vi "Cache.Result.ComponentGet.vi"(7 "Idx":i32, 8 "error in (no error)":errorcluster, 10 "ProdComp in":T1) -> (0 "error out":errorcluster, 1 "Found":bool, 2 "ProdComp out":T1)   [LabVIEW 2016]
uses:
  Cache.ProductComponent.Data.ctl
  Tools/EventLog/EventLog.EventSource.ctl
  Tools/Translator/Translator.Message.ctl
  Tools/EventLog/EventLog.EventLevel.ctl
  Tools/EventLog/EventLog.New(array).vi
  Global/ApplicationGlobal.vi
  Tools/EventLog/EventLog.Buffer.vi
  Tools/EventLog/EventLog.File.ReadWrite.vi
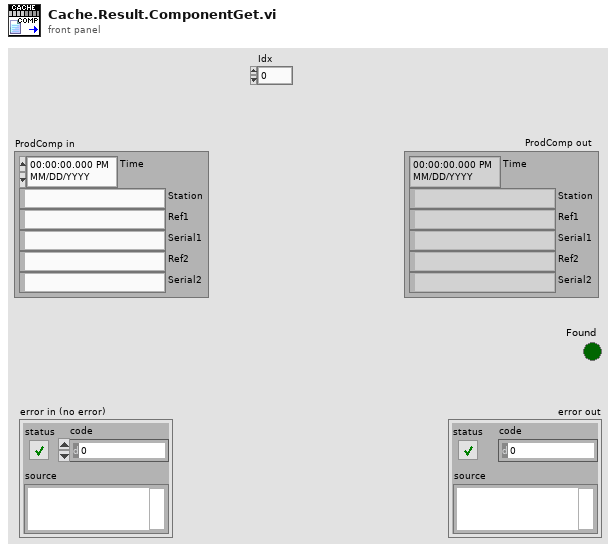
[diagram p1: front panel]
types:
  T1 = typedef "Cache.ProductComponent.Data.ctl" = cluster{"Time":timestamp, "Station":string, "Ref1":string, "Serial1":string, "Ref2":string, "Serial2":string}
  T2 = typedef "EventLog.EventLevel.ctl" = enum8{"Debug", "Info", "Warning", "Error"}
  T3 = typedef "Translator.Message.ctl" = enum16{"-", "Event confirmed", "Log out", "Log in", "Shutdown", "Cancel", "Start", "Continue", "Stop", "On", "Off", "OK", "NOK", "NOK %s", "This", "Prev", "Home", "Work", "In progress...", "Missing", "Empty", "Hardware failure", "Initial", "Error %d >> %s", "Error %d >> %s >> %s", "Starting %s", "Quitting %s", "Configured", "Initializing", "Quitting", "Loading", "Running %s", "Stopped", "Summary", "Do you want to continue?", "Do you want to exit?", "Log out?", "System", "All", "IDLE", "Translating...%s", "Not found", "Alarm %s", "Run", "Skip", "Abort", "Repeat", "Please wait...", "Database disconnected", "Login to database successful", "Login to database failed: %d; %s", "Get process step data for %s", "Changeover off", "Changeover into %s", "Product %s | %s found in cache with status %d at previous station", "Product %s | %s found in database with status %d at previous station", "Product %s | %s not found in cache at previous station", "Product %s | %s not found in database at previous station", "Product %s | %s found in cache with status %d at this station (%d repetion)", "Product %s | %s found in database with status %d at this station (%d repetition)", "Product %s | %s not found in cache at this station", "Product %s | %s not found in database at this station", "Product %s | %s found in cache for component %s | %s", "Product %s | %s found in database for component %s | %s", "Product not found in cache for component %s | %s", "Product not found in database for component %s | %s", "Product %s | %s connected with component %s | %s (cache)", "Product %s | %s connected with component %s | %s (database)", "New data for %s | %s (cache)", "New data for %s | %s (database)", "File %s moved (cache)", "File %s deleted (cache)", "Msg %d >> %s", "PLC LifeBit Failure", "Reconnecting DB", "Reconnecting PLC", "Free disk space is below 1GB - contact technician", "Unable to check product status", "Product %s SN %s checked in DB"}
  T4 = typedef "EventLog.EventSource.ctl" = enum16{"All", "Gui", "Cache", "PLC1", "PLC2", "PLC3", "DB", "DB01", "DB02", "DB03", "DB04", "DB05", "DB06", "DB07", "DB08", "DB09", "DB10", "DB11", "DB12", "DB13", "DB14", "DB15", "DB16"}
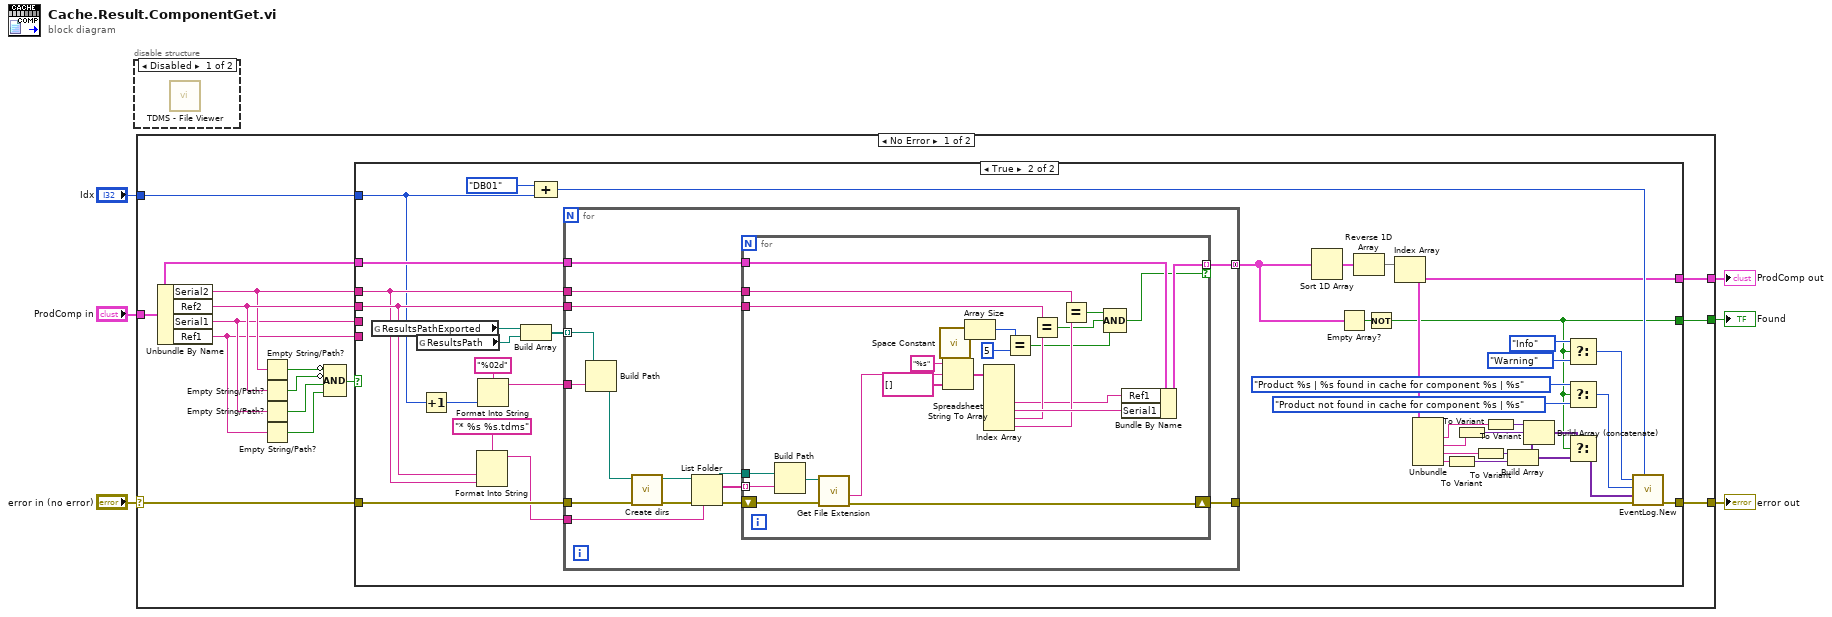
[diagram p0: block diagram]
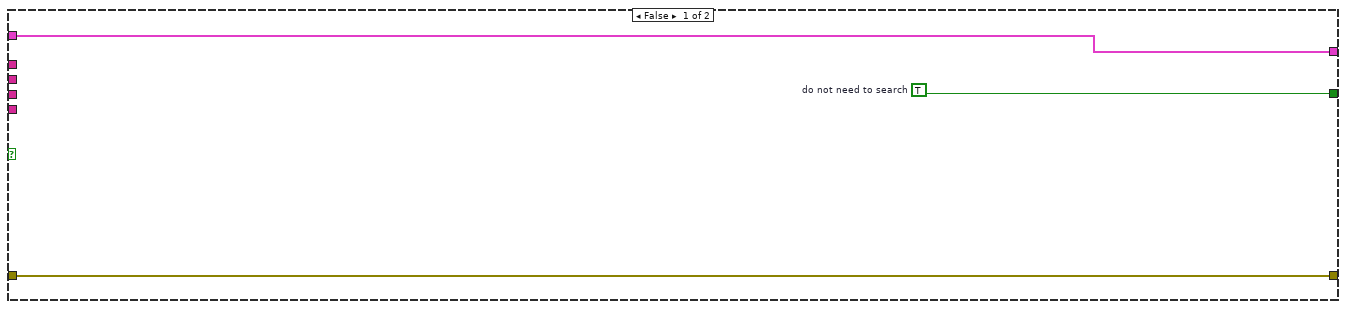
[diagram p2: hidden frame]
diagram:
  n1 = disable-structure shown="Disabled" {
    frame Disabled {
      n2 = call <vilib>:"TDMS - File Viewer.vi"() -> ()  [unwired: 6 in, 2 out]
    }
    frame Enabled {
    }
  }
  n3 = case shown="No Error" "error in (no error)" {
    selector: "error in (no error)" -> [w9 w104]
    tunnel: [w21 w104] -> w6
    tunnel: "ProdComp in" -> [w11 w103]
    tunnel: [w10 w103] -> w3
    tunnel: [w8 _] -> w2
    tunnel: "Idx" -> [w7 _]
    frame No Error {
      n4 = Unbundle By Name(w11) -> ("Serial2"=w19:string, "Ref2"=w20:string, "Serial1"=w18:string, "Ref1"=w17:string)
      n5 = Empty String/Path?(string/path=w19) -> (empty?=w16:bool)
      n6 = Empty String/Path?(string/path=w20) -> (empty?=w15:bool)
      n7 = Empty String/Path?(string/path=w18) -> (empty?=w14:bool)
      n8 = Empty String/Path?(string/path=w17) -> (empty?=w13:bool)
      n9 = Compound Arithmetic op=AND(invert w16, invert w15, w14, w13) -> (w12:bool)
      n10 = case shown="True" w12 {
        tunnel: [w24 w56] -> w21
        tunnel: w9 -> [w24 w63]
        tunnel: w20 -> [_ w34]
        tunnel: w19 -> [_ w33]
        tunnel: w18 -> [_ _]
        tunnel: w17 -> [_ _]
        tunnel: w11 -> [w23 w64]
        tunnel: [w23 w52] -> w10
        tunnel: [w22 w39] -> w8
        tunnel: w7 -> [_ w26]
        frame False {
          w22 = TRUE  # do not need to search
        }
        frame True {
          n11 = global read "ApplicationGlobal.vi" "ResultsPathExported"() -> (w32:path)
          n12 = global read "ApplicationGlobal.vi" "ResultsPath"() -> (w31:path)
          n13 = Increment(x=w26) -> (x+1=w25:i32)
          n14 = Format Into String(format string="* %s %s.tdms", w34, w33) -> (resulting string=w27:string)  [unwired: 2 in, 1 out]
          n15 = Format Into String(format string="%02d", w25) -> (resulting string=w28:string)  [unwired: 2 in, 1 out]
          n16 = Build Array(w32, w31) -> (w30:path[])
          n17 = Compound Arithmetic op=ADD(EventLog.EventSource."DB01" ("Source (All)"), w26) -> (w55:i32)
          n18 = for {
            tunnel: [w67] -> w57
            tunnel: w33 -> [w66]
            tunnel: w34 -> [w65]
            tunnel: w64 -> [w78]
            tunnel: w63 -> [w74]
            tunnel: w30 -> [w76] mode=indexing
            tunnel: [w77] -> w60 mode=concatenating
            tunnel: w28 -> [w75]
            tunnel: w27 -> [w72]
            n19 = Build Path(base path=w76, name or relative path=w75) -> (appended path=w69:path)
            n20 = call "Create dirs.vi"("error in (no error)"=w74, "deepest dir"=w69) -> ("error"=w73:errorcluster)  [unwired: 9 in]
            n21 = List Folder(path=w69, pattern=w72, error in=w73) -> (path out=w68:path, filenames=w70:string[], error out=w71:errorcluster)  [unwired: 1 in, 1 out]
            n22 = for {
              tunnel: w78 -> [w102]
              tunnel: [w101] -> w77 mode=indexing if=w81
              tunnel: w68 -> [w99]
              tunnel: w70 -> [w98] mode=indexing
              shift-right: [w96] -> w67
              shift-left: w71 -> [w100]
              tunnel: w66 -> [w79]
              tunnel: w65 -> [w80]
              n23 = Build Path(base path=w99, name or relative path=w98) -> (appended path=w97:path)
              n24 = call <vilib>:"Get File Extension.vi"("error in (no error)"=w100, "file"=w97) -> ("error out"=w96:errorcluster, "filename without extension"=w95:string)  [unwired: 5 in, 3 out]
              n25 = call <vilib>:"Space Constant.vi"() -> ("String"=w92:string)
              n26 = Spreadsheet String To Array(delimiter (Tab)=w92, format string="%s", spreadsheet string=w95, array type (2D Dbl)=string[] []) -> (array=w90:string[])
              n27 = Array Size(array=w90) -> (size(s)=w89:i32)
              n28 = Index Array(array=w90) -> (element #3=w85:string, element #4=w91:string, element #5=w87:string, element #6=w86:string)  [unwired: 6 in, 2 out]
              n29 = Equal?(x=w89, y=5) -> (x = y?=w82:bool)
              n30 = Equal?(x=w80, y=w87) -> (x = y?=w83:bool)
              n31 = Equal?(x=w79, y=w86) -> (x = y?=w84:bool)
              n32 = Compound Arithmetic op=AND(w84, w83, w82) -> (w81:bool)
              n33 = Bundle By Name(cluster=w102, "Ref1"=w85, "Serial1"=w91) -> (w101:T1)
            }
          }
          n34 = Sort 1D Array(array=w60) -> (sorted array=w62:T1[])
          n35 = Empty Array?(array=w60) -> (empty?=w59:bool)
          n36 = Reverse 1D Array(array=w62) -> (reversed array=w61:T1[])
          n37 = Not(x=w59) -> (.not. x?=w39:bool)
          n38 = Index Array(array=w61) -> (element=w52:T1)  [unwired: 1 in]
          n39 = Unbundle(w52) -> ("Ref1"=w37:string, "Serial1"=w38:string, "Ref2"=w50:string, "Serial2"=w51:string)  [unwired: 2 out]
          n40 = To Variant(anything=w51) -> (Variant=w47:variant)
          n41 = To Variant(anything=w38) -> (Variant=w54:variant)
          n42 = To Variant(anything=w50) -> (Variant=w48:variant)
          n43 = To Variant(anything=w37) -> (Variant=w53:variant)
          n44 = Build Array(w48, w47) -> (w36:variant[])
          n45 = Build Array (concatenate)(w53, w54, w36) -> (w49:variant[])
          n46 = Select(t=EventLog.EventLevel."Info" ("Level (Info)"), s=w39, f=EventLog.EventLevel."Warning" ("Level (Info)")) -> (s? t:f=w40:T2)
          n47 = Select(t=Translator.Message."Product %s | %s found in cache for component %s | %s" ("Message (-)"), s=w39, f=Translator.Message."Product not found in cache for component %s | %s" ("Message (-)")) -> (s? t:f=w44:T3)
          n48 = Select(t=w49, s=w39, f=w36) -> (s? t:f=w43:variant[])
          n49 = call-poly "EventLog.New.vi"("Source (All)"=w55, "error in (no error)"=w57, "Arguments"=w43, "Message (-)"=w44, "Level (Info)"=w40) -> ("error out"=w56:errorcluster)  [unwired: 5 in, 1 out]
        }
      }
    }
    frame Error {
    }
  }
  "error out" <- w6
  "ProdComp out" <- w3
  "Found" <- w2
